vi "Build Async Payload.vi"(8 "error in (no error)":errorcluster, 10 "Async Pointers":T2 {"LP Async Data Addresses" format="%04x"; "LP Async Control Addresses" format="%04x"; "HP Async Data Addresses" format="%04x"; "HP Async Control Addresses" format="%04x"}, 11 "Async Message in":refnum<class "Async Message.lvclass">) -> (0 "error out":errorcluster, 2 "Async Payload":T1 {"Trigger Command" format="%04x"; "Data" format="%04x"; "Data Address" format="%04x"; "Configuration" format="%04x"; "Configuration Address" format="%04x"}, 3 "Async Message out":refnum<class "Async Message.lvclass">)   [LabVIEW 2020, in "BCI-1553 API.lvlib" / "Async Message.lvclass"]
doc: "<DO NOT CALL>\n\nBuilds the data payload that will need to be sent down to the Holt IC by the caller."
uses:
  Async Message.lvclass
  TypeDefs/Async Message Pointers.ctl
  TypeDefs/Async Payload.ctl
  Async Message.lvclass/Async Message.ctl
  BCI-1553 API.lvlib
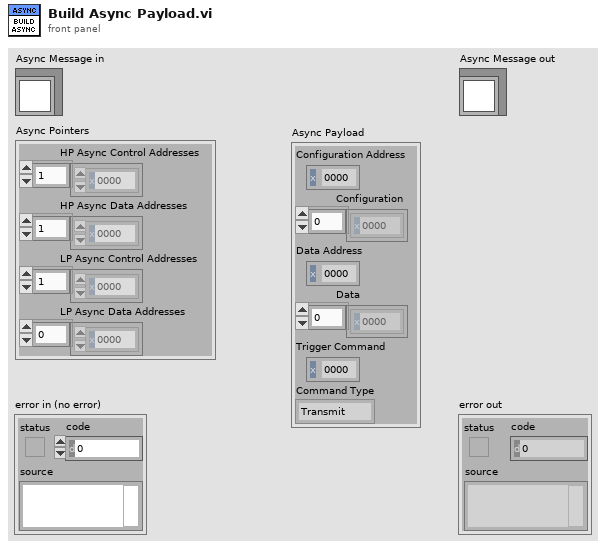
[diagram p1: front panel]
types:
  T1 = typedef "BCI-1553 API.lvlib/Async Payload.ctl" = cluster{"Configuration Address":u16, "Configuration":u16[], "Data Address":u16, "Data":u16[], "Trigger Command":u16, "Command Type":enum16{"Transmit", "Receive"}}
  T2 = typedef "BCI-1553 API.lvlib/Async Message Pointers.ctl" = cluster{"HP Async Control Addresses":u16[], "HP Async Data Addresses":u16[], "LP Async Control Addresses":u16[], "LP Async Data Addresses":u16[]}
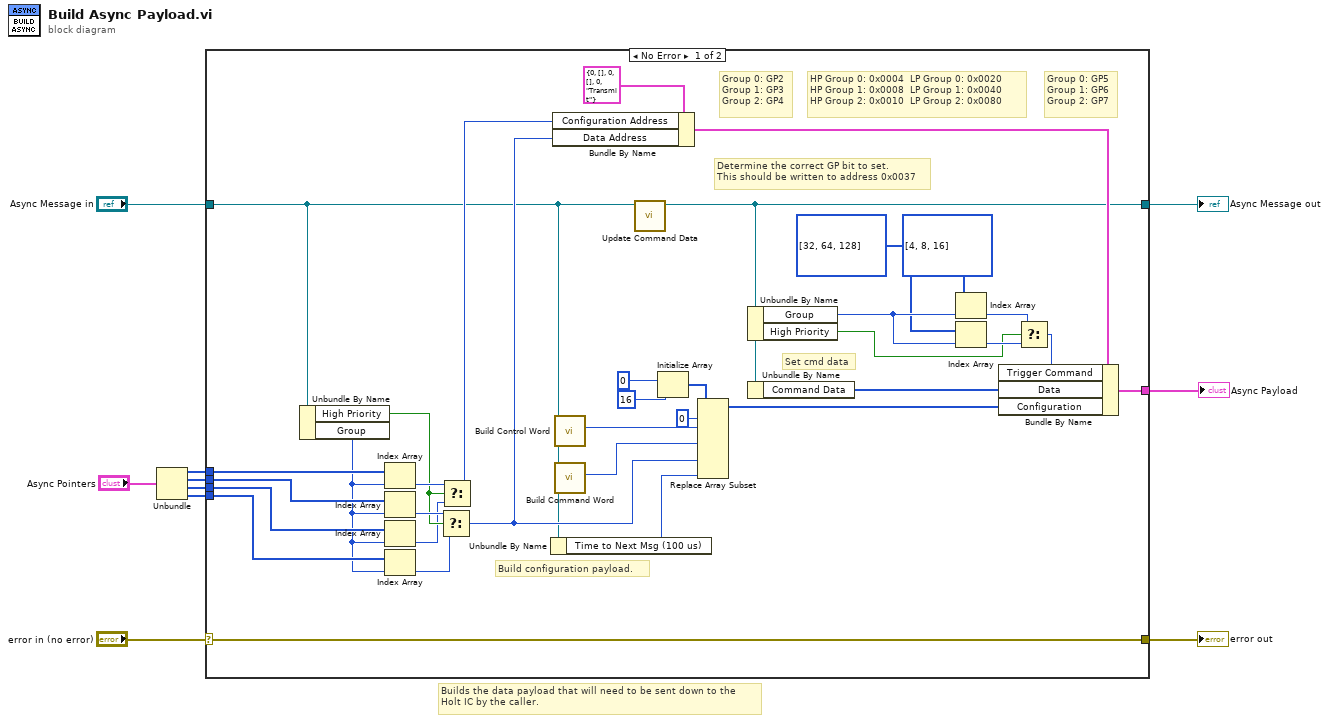
[diagram p0: block diagram]
diagram:
  # "Builds the data payload that will need to be sent down to the\nHolt IC by the caller."
  n1 = Unbundle("Async Pointers") -> ("HP Async Control Addresses"=w3:u16[], "HP Async Data Addresses"=w5:u16[], "LP Async Control Addresses"=w2:u16[], "LP Async Data Addresses"=w4:u16[])
  n2 = case shown="No Error" "error in (no error)" {
    selector: "error in (no error)" -> [w44 w46]
    tunnel: [w44 w46] -> w9
    tunnel: [w11 w45] -> w7
    tunnel: "Async Message in" -> [w12 w45]
    tunnel: w5 -> [w42 _]
    tunnel: w4 -> [w43 _]
    tunnel: w3 -> [w30 _]
    tunnel: w2 -> [w31 _]
    tunnel: [w22 _] -> w1
    frame No Error {
      # "Group 0: GP5\nGroup 1: GP6\nGroup 2: GP7"
      # "Group 0: GP2\nGroup 1: GP3\nGroup 2: GP4"
      # "HP Group 0: 0x0004  LP Group 0: 0x0020  \nHP Group 1: 0x0008  LP Group 1: 0x0040  \nHP Group 2: 0x0010  LP Group 2: 0x0080"
      # "Determine the correct GP bit to set.\nThis should be written to address 0x0037"
      # "Set cmd data"
      # "Build configuration payload."
      n3 = Unbundle By Name(w12) -> ("High Priority"=w27:bool, "Group"=w29:i32)
      n4 = Index Array(array=w30, index=w29) -> (element=w28:u16)
      n5 = Index Array(array=w42, index=w29) -> (element=w41:u16)
      n6 = Index Array(array=w31, index=w29) -> (element=w26:u16)
      n7 = Index Array(array=w43, index=w29) -> (element=w40:u16)
      n8 = Select(t=w41, s=w27, f=w40) -> (s? t:f=w13:u16)
      n9 = Select(t=w28, s=w27, f=w26) -> (s? t:f=w25:u16)
      n10 = Unbundle By Name(w12) -> ("Time to Next Msg (100 us)"=w33:u16)
      n11 = Bundle By Name(cluster=T1 {"Configuration Address"=0, "Configuration"=[], "Data Address"=0, "Data"=[], "Trigger Command"=0, "Command Type"=enum."Transmit"} ("Async Payload"), "Configuration Address"=w25, "Data Address"=w13) -> (w24:T1)
      n12 = call-dynamic "Build Control Word.vi"("Async Message in"=w12) -> ("Control Word"=w35:u16)  [unwired: 9 in, 1 out]
      n13 = call-dynamic "Build Command Word.vi"("Async Message in"=w12) -> ("Command Word"=w34:u16)  [unwired: 9 in, 1 out]
      n14 = call-dynamic "Update Command Data.vi"("Async Message in"=w12) -> ("Async Message out"=w11:refnum<class "Async Message.lvclass">)  [unwired: 9 in, 1 out]
      n15 = Initialize Array(u16 0 ("Command Word"), 16 ("dimension size")) -> (w37:u16[])
      n16 = Replace Array Subset(array=w37, new element #1=w35, index #1=0 ("index"), new element #2=w34, new element #3=w13, new element #4=w33) -> (w23:u16[])  [unwired: 3 in]
      n17 = Unbundle By Name(w11) -> ("Group"=w19:i32, "High Priority"=w14:bool)
      n18 = Unbundle By Name(w11) -> ("Command Data"=w21:u16[])
      n19 = Index Array(array=u16[] [4, 8, 16] ("Command Word"), index=w19) -> (element=w17:u16)
      n20 = Index Array(array=u16[] [32, 64, 128] ("Command Word"), index=w19) -> (element=w16:u16)
      n21 = Select(t=w17, s=w14, f=w16) -> (s? t:f=w15:u16)
      n22 = Bundle By Name(cluster=w24, "Trigger Command"=w15, "Data"=w21, "Configuration"=w23) -> (w22:T1)
    }
    frame Error {
    }
  }
  "error out" <- w9
  "Async Message out" <- w7
  "Async Payload" <- w1
